vi "TSCAN ChannelCount.vi"(0 "路径输入":path, 5 "使用通道数量":i32(ring)=1 items=["1通道"=1, "2通道"=2, "3通道"=3, "4通道"=4, "5通道"=5], 11 "错误输入（无错误）":errorcluster) -> (4 "路径输出":path, 6 "CANCount":i32, 15 "错误输出":errorcluster)   [LabVIEW 2013]
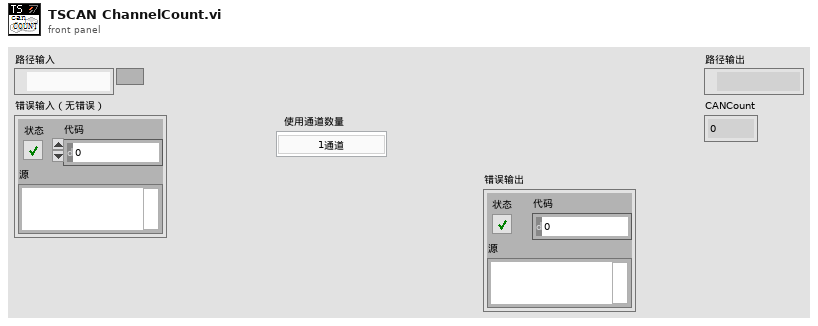
[diagram p1: front panel]
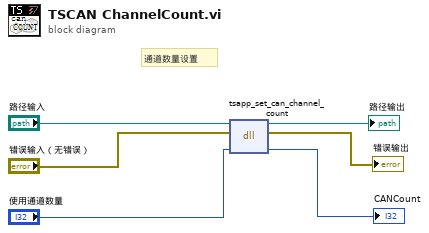
[diagram p0: block diagram]
diagram:
  # "通道数量设置"
  n1 = dll-call lib="PTH1Habs CUsers\nAdministratorDesktopTS_Can通讯PathTSMaster.dll" fn="tsapp_set_can_channel_count"(path in="路径输入", error in="错误输入（无错误）", "Aount"="使用通道数量") -> (path out=→"路径输出":path, error out=→"错误输出":errorcluster, "Aount"=→"CANCount":i32)  [unwired: 2 in]
